vi "JSON_Formats.vi"() -> ()   [LabVIEW 2020]
panel:
  in  "Write text 2":refnum<vi>
  in  "Woody":refnum<vi>
  in  "Table Control":string[][](table)=[["PUT localhost:6000/Code", "{\"Code\":\"import os \\n\"}", "Success"], ["GET localhost:6000/REPL", "", "{\"REPL\":\"import os \\n\"}"], ["GET localhost:6000/state", "", "{\"Connection\":\"COM3\", \"Connected?\":true}"], ["PUT localhost:6000/Save", "{\"Name\":\"test.py\", \"Code\":\"import os \\n\"}", "Success"]]
  in  "Save":cluster{"fileName":string, "Code":string}
  in  "state":cluster{"Connection":string, "Connected?":bool}={"Connection"="", "Connected?"=TRUE}
  in  "REPL":cluster{"REPL":string}
  in  "Code":cluster{"Code":string}
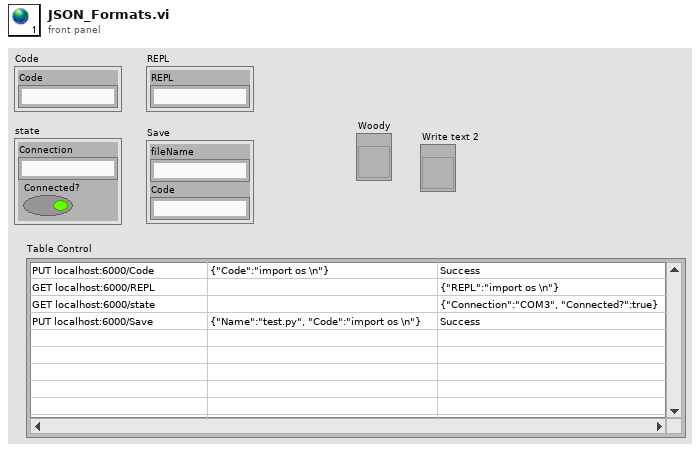
[diagram p1: front panel]
diagram:
